vi "Load Config.vi"(8 "error in (no error)":errorcluster, 10 "Storage":refnum<class "Config Storage.lvclass">, 11 "Config Manager in":refnum<class "Config Manager.lvclass">) -> (0 "error out":errorcluster, 3 "Config Manager out":refnum<class "Config Manager.lvclass">)   [LabVIEW 2020, in "CDM-Config.lvlib" / "Config Manager.lvclass"]
uses:
  Config Manager.lvclass
  Config Storage/Config Storage.lvclass
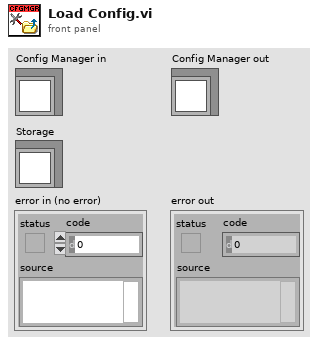
[diagram p1: front panel]
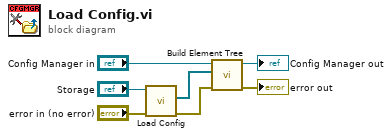
[diagram p0: block diagram]
diagram:
  n1 = call-dynamic "Load Config.vi"("error in (no error)"="error in (no error)", "Config Storage in"="Storage") -> ("error out"=w2:errorcluster, "Elements"=w3:refnum<class "Config Element.lvclass">[])  [unwired: 7 in, 1 out]
  n2 = call "Build Element Tree.vi"("error in (no error)"=w2, "Elements in"=w3, "Config Manager in"="Config Manager in") -> ("error out"=→"error out":errorcluster, "Config Manager out"=→"Config Manager out":refnum<class "Config Manager.lvclass">)  [unwired: 7 in]
